vi "FGV Register and Unregister.vi"() -> (4 "response message":string[](array[string]), 6 "response message":string[](array[string]), 8 "response message":string[](array[string]), 10 "response message":string[](array[string]), 15 "response message":string[](array[string]))   [LabVIEW 2017, in "testcase-Broadcast Registry.lvclass"]
uses:
  testcase-Broadcast Registry.lvclass
  src/user.lib/_NEVSTOP/Communicable State Machine(CSM)/_Support/FGV-BroadcastRegistry/Operation-BroadcastRegistry.ctl
  src/user.lib/_NEVSTOP/Communicable State Machine(CSM)/Communicable State Machine.lvlib
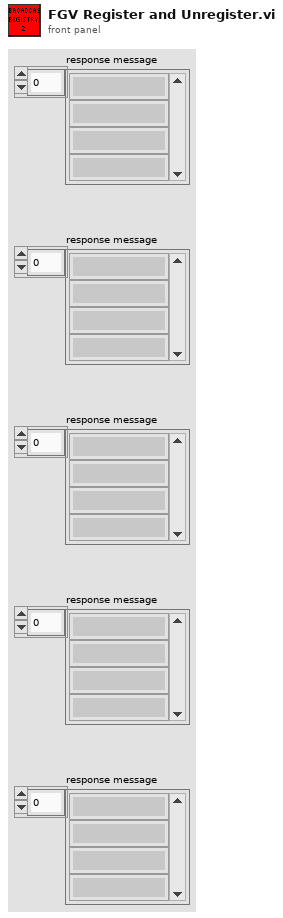
[diagram p1: front panel]
types:
  T1 = typedef "Communicable State Machine.lvlib/Operation-BroadcastRegistry.ctl" = enum16{"Delete Source Module", "Delete Target Module", "Remove Module", "Register", "Unregister", "Check", "List Status", "List Entries", "List Status Of Source", "Drop", "Register As Status", "Register As Interrupt"}
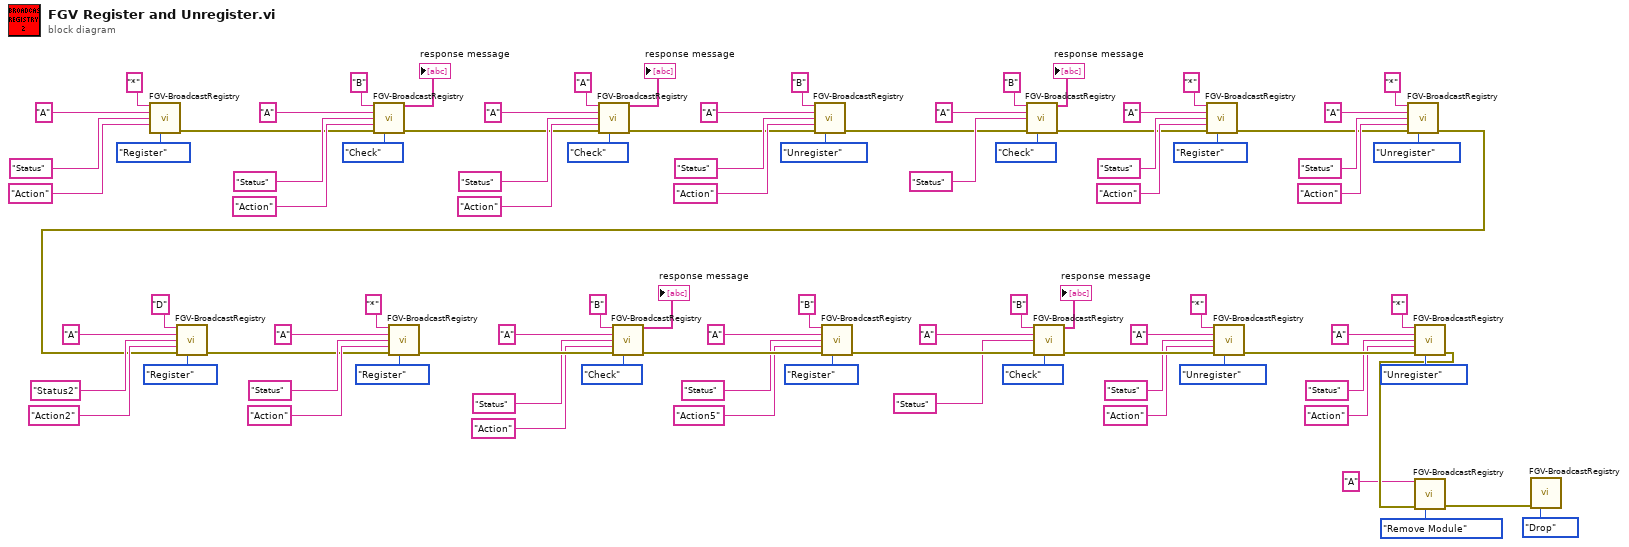
[diagram p0: block diagram]
diagram:
  n1 = call "FGV-BroadcastRegistry.vi"("Source"="*", "Target"="A" ("Dest"), "Status"="Status" ("Message"), "API"="Action" ("Response Message In"), "Operation"=Operation-BroadcastRegistry."Register") -> ("error out"=w81:errorcluster)  [unwired: 8 in, 2 out]
  n2 = call "FGV-BroadcastRegistry.vi"("Source"="B", "Target"="A" ("Dest"), "Status"="Status" ("Message"), "API"="Action" ("Response Message In"), "Error In"=w81, "Operation"=Operation-BroadcastRegistry."Check") -> ("Response Message"=→"response message":string[], "error out"=w4:errorcluster)  [unwired: 7 in, 1 out]
  n3 = call "FGV-BroadcastRegistry.vi"("Source"="A", "Target"="A" ("Dest"), "Status"="Status" ("Message"), "API"="Action" ("Response Message In"), "Error In"=w4, "Operation"=Operation-BroadcastRegistry."Check") -> ("Response Message"=→"response message":string[], "error out"=w3:errorcluster)  [unwired: 7 in, 1 out]
  n4 = call "FGV-BroadcastRegistry.vi"("Source"="B", "Target"="A" ("Dest"), "Status"="Status" ("Message"), "API"="Action" ("Response Message In"), "Error In"=w3, "Operation"=Operation-BroadcastRegistry."Unregister") -> ("error out"=w69:errorcluster)  [unwired: 7 in, 2 out]
  n5 = call "FGV-BroadcastRegistry.vi"("Source"="B", "Target"="A" ("Dest"), "Status"="Status" ("Message"), "Error In"=w69, "Operation"=Operation-BroadcastRegistry."Check") -> ("Response Message"=→"response message":string[], "error out"=w63:errorcluster)  [unwired: 8 in, 1 out]
  n6 = call "FGV-BroadcastRegistry.vi"("Source"="*", "Target"="A" ("Dest"), "Status"="Status" ("Message"), "API"="Action" ("Response Message In"), "Error In"=w63, "Operation"=Operation-BroadcastRegistry."Register") -> ("error out"=w57:errorcluster)  [unwired: 7 in, 2 out]
  n7 = call "FGV-BroadcastRegistry.vi"("Source"="*", "Target"="A" ("Dest"), "Status"="Status" ("Message"), "API"="Action" ("Response Message In"), "Error In"=w57, "Operation"=Operation-BroadcastRegistry."Unregister") -> ("error out"=w15:errorcluster)  [unwired: 7 in, 2 out]
  n8 = call "FGV-BroadcastRegistry.vi"("Source"="D", "Target"="A" ("Dest"), "Status"="Status2" ("Message"), "API"="Action2" ("Response Message In"), "Error In"=w15, "Operation"=Operation-BroadcastRegistry."Register") -> ("error out"=w14:errorcluster)  [unwired: 7 in, 2 out]
  n9 = call "FGV-BroadcastRegistry.vi"("Source"="*", "Target"="A" ("Dest"), "Status"="Status" ("Message"), "API"="Action" ("Response Message In"), "Error In"=w14, "Operation"=Operation-BroadcastRegistry."Register") -> ("error out"=w31:errorcluster)  [unwired: 7 in, 2 out]
  n10 = call "FGV-BroadcastRegistry.vi"("Source"="B", "Target"="A" ("Dest"), "Status"="Status" ("Message"), "API"="Action" ("Response Message In"), "Error In"=w31, "Operation"=Operation-BroadcastRegistry."Check") -> ("Response Message"=→"response message":string[], "error out"=w38:errorcluster)  [unwired: 7 in, 1 out]
  n11 = call "FGV-BroadcastRegistry.vi"("Source"="B", "Target"="A" ("Dest"), "Status"="Status" ("Message"), "API"="Action5" ("Response Message In"), "Error In"=w38, "Operation"=Operation-BroadcastRegistry."Register") -> ("error out"=w44:errorcluster)  [unwired: 7 in, 2 out]
  n12 = call "FGV-BroadcastRegistry.vi"("Source"="B", "Target"="A" ("Dest"), "Status"="Status" ("Message"), "Error In"=w44, "Operation"=Operation-BroadcastRegistry."Check") -> ("Response Message"=→"response message":string[], "error out"=w50:errorcluster)  [unwired: 8 in, 1 out]
  n13 = call "FGV-BroadcastRegistry.vi"("Source"="*", "Target"="A" ("Dest"), "Status"="Status" ("Message"), "API"="Action" ("Response Message In"), "Error In"=w50, "Operation"=Operation-BroadcastRegistry."Unregister") -> ("error out"=w56:errorcluster)  [unwired: 7 in, 2 out]
  n14 = call "FGV-BroadcastRegistry.vi"("Source"="*", "Target"="A" ("Dest"), "Status"="Status" ("Message"), "API"="Action" ("Response Message In"), "Error In"=w56, "Operation"=Operation-BroadcastRegistry."Unregister") -> ("error out"=w12:errorcluster)  [unwired: 7 in, 2 out]
  n15 = call "FGV-BroadcastRegistry.vi"("Source"="A" ("Dest"), "Error In"=w12, "Operation"=Operation-BroadcastRegistry."Remove Module") -> ("error out"=w1:errorcluster)  [unwired: 10 in, 2 out]
  n16 = call "FGV-BroadcastRegistry.vi"("Error In"=w1, "Operation"=Operation-BroadcastRegistry."Drop") -> ()  [unwired: 11 in, 3 out]
